vi "PolarizationSimulation_Final.vi"() -> ()   [LabVIEW 2020]
uses:
  Integrated ANN/Sub-VIs/Adam_data.ctl
  <vilib>/Utility/xml.llb/Read From XML File(string).vi
  <vilib>/Utility/xml.llb/Write to XML File(string).vi
  <vilib>/Analysis/NI_AALBase.lvlib
panel:
  out "NN Graph":cluster{dbl[], dbl[]}(graph)
  in  "Regularization":T1
  in  "Batch Size":i16
  out "NN Loss":dbl(graph)
  in  "Loss Function":enum16{"MSE", "MAE"}(ring)
  in  "Parameters File Path":path
  out "NN Error":dbl
  in  "Training?":bool
  out "NN Output":dbl
  in  "Speed\nMultiplier":dbl=1.0
  in  "AFP On":bool
  in  "AFP Efficiency":dbl=0.9 min=0.0 max=1.0 step=0.01
  in  "AFP Control":cluster{i32, i32}(slide)={200, 230} scale=0.0..500.0
  out "lower R-value AFP":dbl
  out "upper R-value AFP":dbl
  in  "STOP":bool
  in  "Microwave Power":dbl=1.0
  in  "Lower Fit\nParameter":dbl=-3.6
  in  "Upper Fit\nParameter":dbl=3.6
  in  "Std Dev Noise":dbl step=0.0001
  out "lower R-value":dbl
  out "upper R-value":dbl
  in  "RF Control":cluster{i32, i32}(slide)={200, 230} scale=0.0..500.0
  out "p":dbl format="%_4g"
  out "r":dbl
  in  "Saturation\nPolarization":dbl=0.8 min=0.0 max=0.99 step=0.01
  out "Reimann \nsum of Q":dbl format="%_4g"
  out "Corrected Data (Q)":cluster{dbl[], dbl[]}(graph)
  in  "Select Target Type":u16(ring)=2 items=["Test Case", "Deuteron"]
  in  "Reset":bool
  out "Total Polarization (P)":cluster{dbl, dbl}(graph)
  in  "Spin Manipulation\nPower Factor":dbl=0.005
  in  "Decay Spin\nManipulation":bool
  out "Reimann\nsum of P":dbl format="%_4g"
  out "Corrected Data (P)":cluster{dbl[], dbl[]}[](graph)
  out "Signal and Fit (P)":cluster{dbl[], "Best Polynomial Fit":dbl[]}[](graph)
  in  "Positive\nPolarization":bool
  in  "Microwave on":bool
  # "Neural Network"
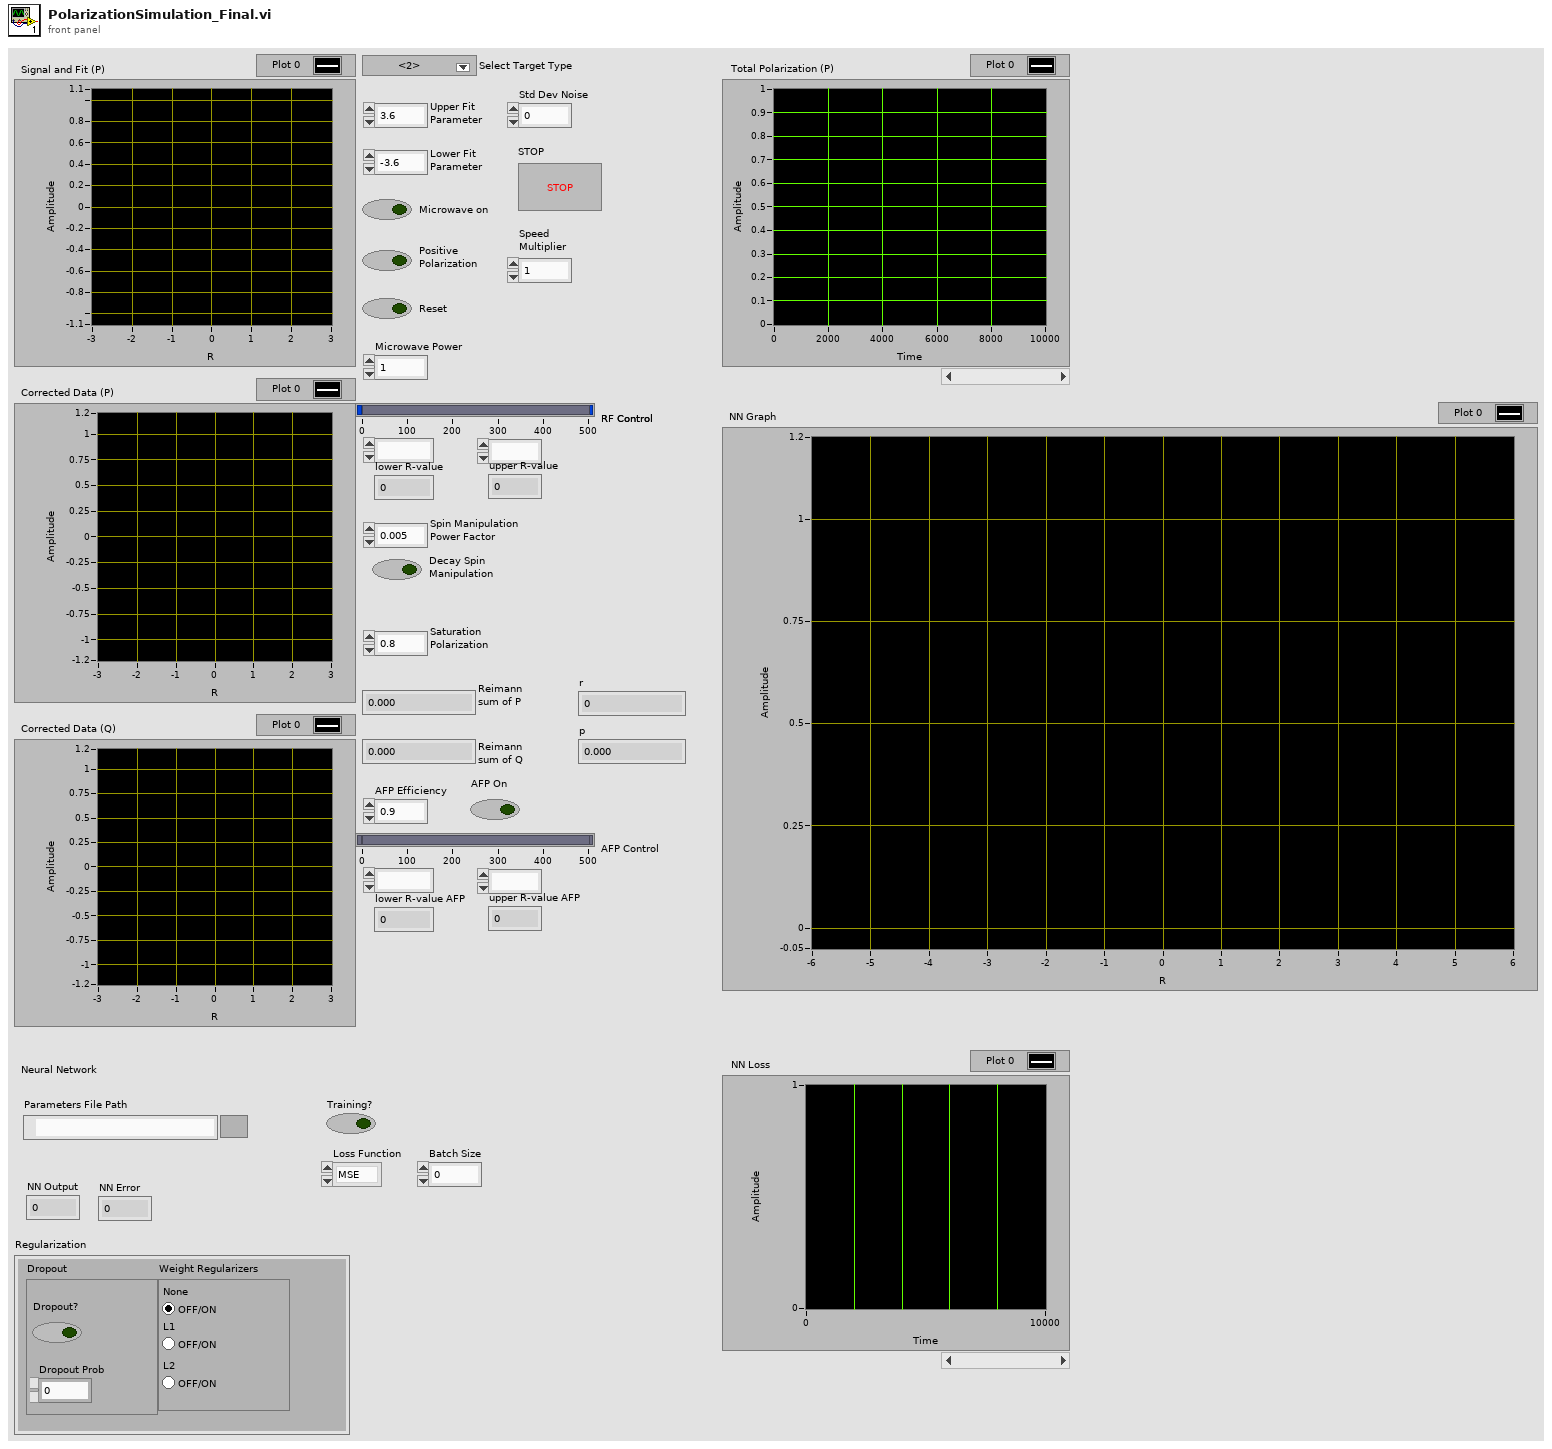
[diagram p1: front panel]
types:
  T1 = cluster{"Dropout":cluster{"Dropout?":bool, "Dropout Prob":dbl}, "Weight Regularizers":enum32{"None", "L1", "L2"}}
  T2 = typedef "Adam_data.ctl" = cluster{"Mw Moments":cluster{"3 ":dbl[], "2":dbl[][], "1":dbl[][]}, "Vw Moments":cluster{"3":dbl[], "2":dbl[][], "1":dbl[][]}, "Mb Moments":cluster{"3":dbl, "2":dbl[], "1":dbl[]}, "Vb Moments":cluster{"3":dbl, "2":dbl[], "1":dbl[]}}
  T3 = cluster{cluster{dbl[][], dbl[]}, cluster{dbl[][], dbl[]}, cluster{dbl[], dbl}}
  T4 = cluster{cluster{"Updated Weights":dbl[][], "Updated Biases":dbl[]}, cluster{"Updated Weights":dbl[][], "Updated Biases":dbl[]}, cluster{"Updated Weights":dbl[], "Updated Biases":dbl}}
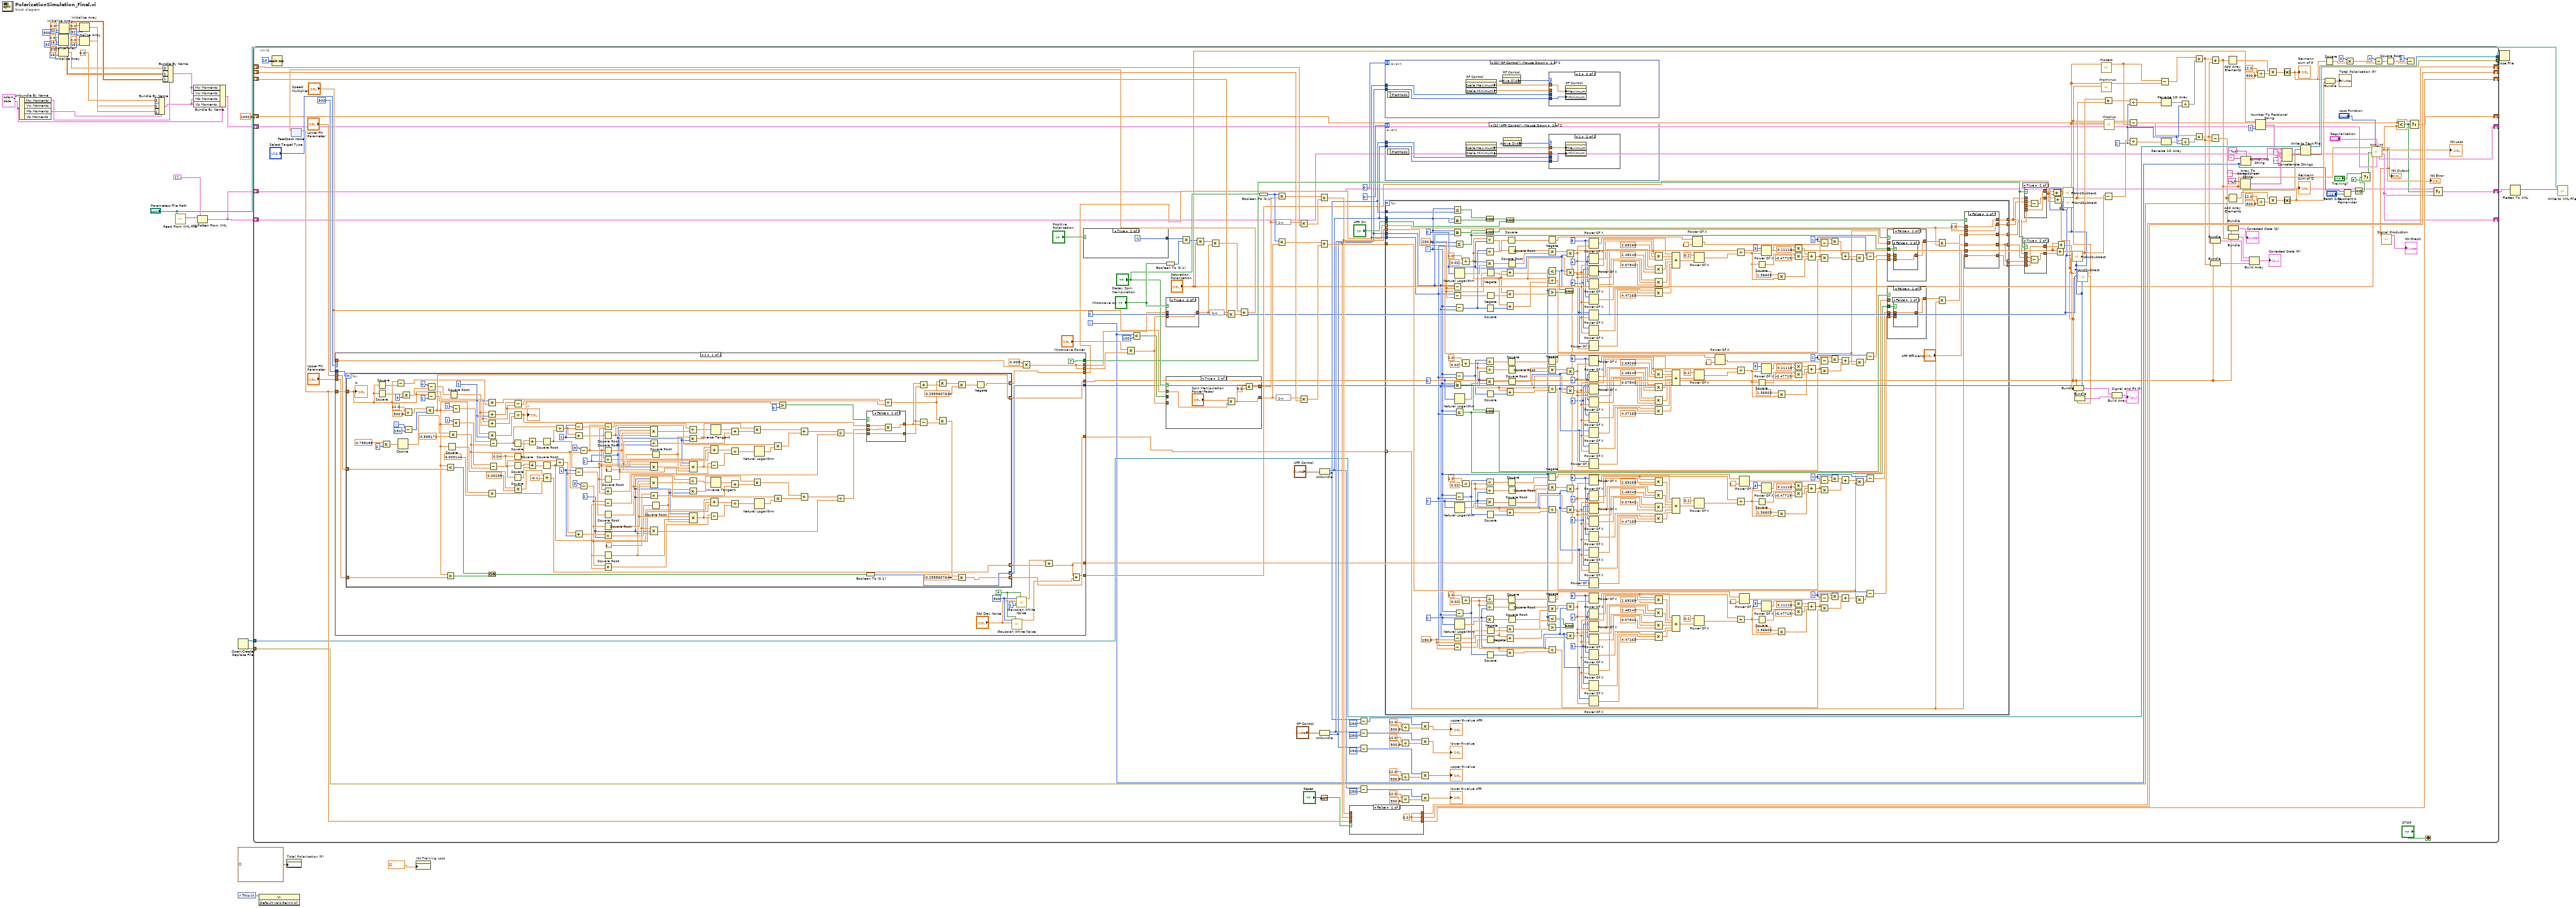
[diagram p0: block diagram]
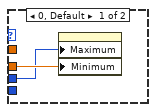
[diagram p2: hidden frame]
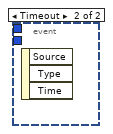
[diagram p3: hidden frame]
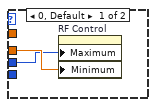
[diagram p4: hidden frame]
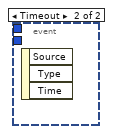
[diagram p5: hidden frame]
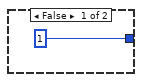
[diagram p6: hidden frame]
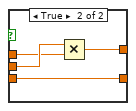
[diagram p7: hidden frame]
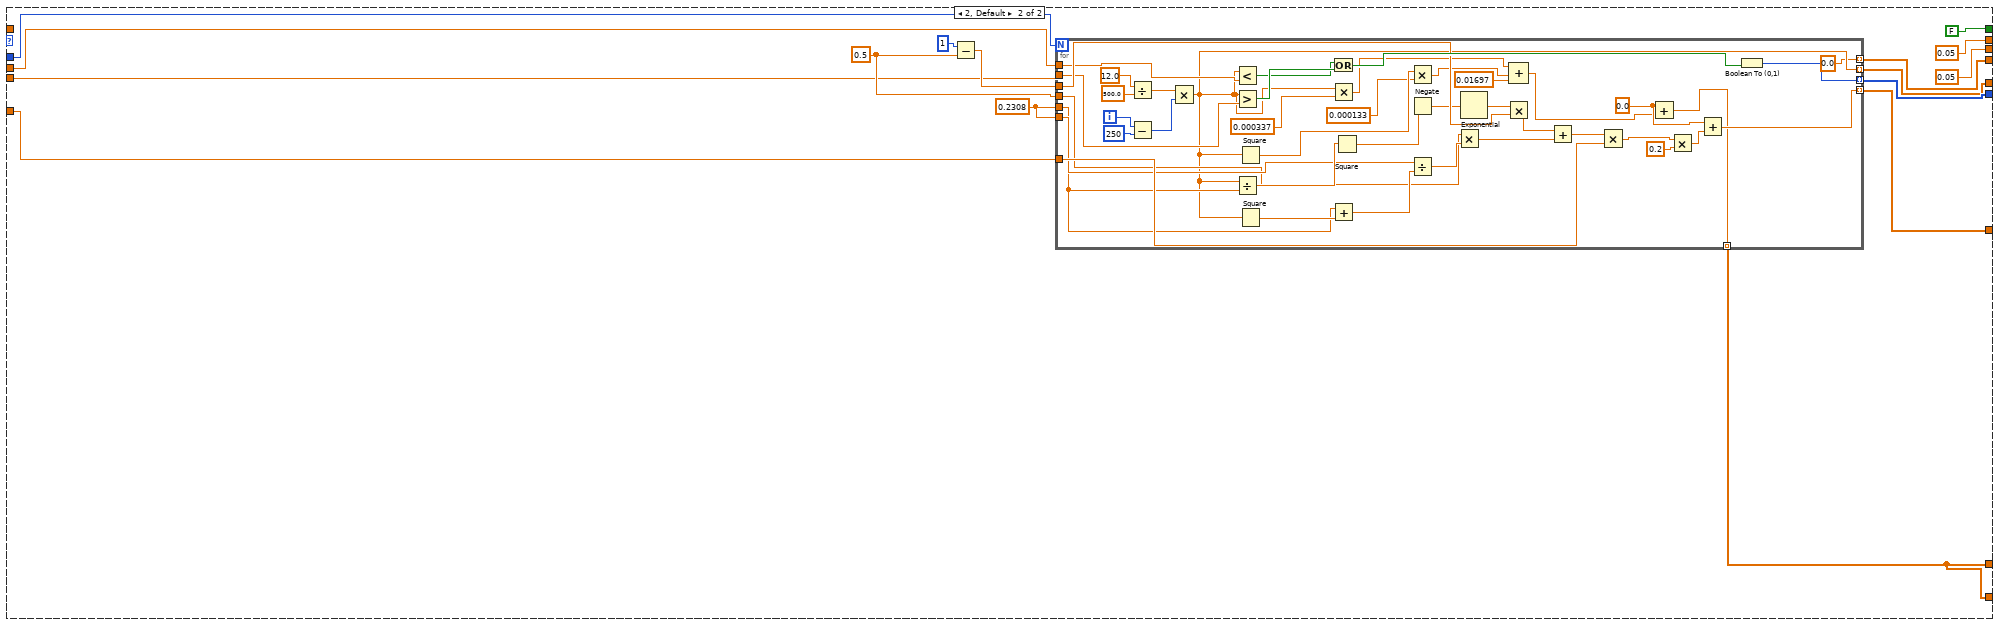
[diagram p8: hidden frame]
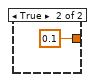
[diagram p10: hidden frame]
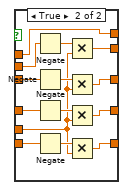
[diagram p15: hidden frame]
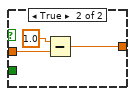
[diagram p17: hidden frame]
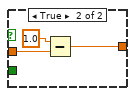
[diagram p19: hidden frame]
diagram:
  w7 = T2 {"Mw Moments"={"3 "=[], "2"=[], "1"=[]}, "Vw Moments"={"3"=[], "2"=[], "1"=[]}, "Mb Moments"={"3"=0.0, "2"=[], "1"=[]}, "Vb Moments"={"3"=0.0, "2"=[], "1"=[]}} ("Adam Data In")
  n1 = Unbundle By Name(w7) -> ("Mw Moments"=w9:cluster{"3 ":dbl[], "2":dbl[][], "1":dbl[][]}, "Mb Moments"=w8:cluster{"3":dbl, "2":dbl[], "1":dbl[]})  [unwired: 2 out]
  n2 = Initialize Array(0.0 ("element"), 16 ("dimension size"), 32 ("dimension size")) -> (w14:dbl[][])
  n3 = Initialize Array(0.0 ("element"), 16 ("dimension size")) -> (w13:dbl[])
  n4 = Initialize Array(0.0 ("element"), 32 ("dimension size"), 500 ("dimension size")) -> (w15:dbl[][])
  n5 = Initialize Array(0.0 ("element"), 16 ("dimension size")) -> (w11:dbl[])
  n6 = Initialize Array(0.0 ("element"), 32 ("dimension size")) -> (w12:dbl[])
  n7 = Bundle By Name(cluster=w8, "3"=0.0 ("element"), "2"=w11, "1"=w12) -> (w5:cluster{"3":dbl, "2":dbl[], "1":dbl[]})
  n8 = Bundle By Name(cluster=w9, "3"=w13, "2"=w14, "1"=w15) -> (w6:cluster{"3 ":dbl[], "2":dbl[][], "1":dbl[][]})
  n9 = call-poly <vilib>:"Read From XML File.vi"("XML File Path"="Parameters File Path") -> ("XML Elements"=w32:string)  [unwired: 8 in, 2 out]
  n10 = Bundle By Name(cluster=w7, "Mw Moments"=w6, "Vw Moments"=w6, "Mb Moments"=w5, "Vb Moments"=w5) -> (w4:T2)
  n11 = Unflatten From XML(xml string=w32, type=T3 {{[], []}, {[], []}, {[], 0.0}}) -> (value=w3:T3)  [unwired: 1 in, 1 out]
  n12 = Open/Create/Replace File() -> (refnum out=w36:refnum<file>, error out=w35:errorcluster)  [unwired: 6 in, 1 out]
  n13 = control-ref of="This VI"() -> (w38:refnum<vi>)
  n14 = while {
    shift-right: [w213] -> _
    shift-left: _ -> [w220]
    shift-right: [w212] -> _
    shift-left: _ -> [w195]
    shift-right: [w190] -> _
    shift-left: _ -> [w189]
    tunnel: w36 -> [w122]
    tunnel: w35 -> [w121]
    tunnel: [w120] -> w34
    tunnel: [w119] -> w33
    shift-right: [w44] -> _
    shift-left: w3 -> [w59]
    shift-right: [w57] -> _
    shift-left: w4 -> [w56]
    shift-right: [w48] -> _
    shift-left: 1000.0 ("Error") -> [w47]
    shift-right: [w43] -> w2
    shift-left: w3 -> [w42]
    i -> [w55]
    stop <- "STOP" stop-if-true
    w172 = 2
    w68 = 2
    n15 = Wait (ms)(milliseconds to wait=10) -> ()  [unwired: 1 out]
    n16 = feedback #1() -> (w199:dbl)  [unwired: 1 in]
    n17 = case shown="1" "Select Target Type" {
      tunnel: [w255 0.05 ("Growth Constant")] -> w204
      tunnel: [w255 0.05 ("Decay Constant")] -> w203
      tunnel: 500 -> [w264 w422]
      tunnel: w199 -> [w267 w421]
      tunnel: "Upper Fit\nParameter" -> [w265 w419]
      tunnel: "Lower Fit\nParameter" -> [w266 w420]
      tunnel: [w262 w417] -> w67
      tunnel: [w252 w416] -> w82
      tunnel: [w263 w418] -> w66
      tunnel: [TRUE FALSE] -> w183
      tunnel: [w253 w412] -> w81
      tunnel: "Speed\nMultiplier" -> [w254 _]
      tunnel: [w248 w411] -> w80
      tunnel: [w250 w411] -> w79
      frame 1 {
        w257 = FALSE
        w259 = 500
        n18 = for {
          N: w264 -> [_]
          tunnel: [w298] -> w262 mode=indexing
          tunnel: [w387] -> w263 mode=indexing
          tunnel: w265 -> [w386]
          tunnel: w266 -> [w385]
          tunnel: [w270] -> w252 mode=indexing
          tunnel: w267 -> [w271]
          tunnel: [w269] -> w253 mode=indexing
          tunnel: [w268] -> w251 mode=indexing
          i -> [w363]
          w285 = 2
          w324 = 1
          w328 = 3.141592653589793
          w322 = 2
          w307 = 0.04
          w360 = 1
          w365 = 3.141592653589793
          w358 = 2
          n19 = Square(x=w271) -> (x^2=w288:dbl)
          n20 = Square(x=w271) -> (x^2=w314:dbl)
          n21 = Multiply(x=0.758188, y=2) -> (x*y=w302:dbl)
          n22 = Subtract(x=w271, y=w288) -> (x-y=w287:dbl)
          n23 = Cosine(x=w302) -> (cos(x)=w305:dbl)
          n24 = Multiply(x=w314, y=3) -> (x*y=w313:dbl)
          n25 = Divide(x=12.0, y=500.0) -> (x/y=w401:dbl)
          n26 = Subtract(x=w363, y=250) -> (x-y=w400:i32)
          n27 = Multiply(x=w401, y=w400) -> (x*y=w298:dbl)
          n28 = Subtract(x=4, y=w313) -> (x-y=w311:dbl)
          n29 = Subtract(x=w271, y=1) -> (x-y=w309:dbl)
          n30 = Less?(x=w298, y=w385) -> (x < y?=w390:bool)
          n31 = Greater?(x=w298, y=w386) -> (0:w389:bool)
          n32 = Square(x=w298) -> (x^2=w300:dbl)
          n33 = Multiply(x=w305, y=0.558171) -> (x*y=w306:dbl)
          n34 = Square Root(x=w311) -> (sqrt(x)=w286:dbl)
          n35 = Subtract(x=1, y=w298) -> (x-y=w395:dbl)
          n36 = Add(x=1, y=w298) -> (x+y=w352:dbl)
          n37 = Multiply(x=w285, y=w287) -> (x*y=w283:dbl)
          n38 = Add(x=w286, y=w285) -> (x+y=w284:dbl)
          n39 = Add(x=w271, y=w286) -> (x+y=w310:dbl)
          n40 = Multiply(x=w309, y=w285) -> (x*y=w293:dbl)
          n41 = Multiply(x=w298, y=0.000144) -> (x*y=w295:dbl)
          n42 = Or(x=w390, y=w389) -> (x .or. y?=w388:bool)
          n43 = Subtract(x=w395, y=w306) -> (x-y=w391:dbl)
          n44 = Subtract(x=w352, y=w306) -> (x-y=w348:dbl)
          n45 = Square(x=w391) -> (x^2=w394:dbl)
          n46 = Square(x=w307) -> (x^2=w393:dbl)
          n47 = Square(x=w307) -> (x^2=w350:dbl)
          n48 = Square(x=w348) -> (x^2=w351:dbl)
          n49 = Subtract(x=w284, y=w271) -> (x-y=w282:dbl)
          n50 = Divide(x=w310, y=w293) -> (x/y=w289:dbl)
          "r" <- w289
          n51 = Multiply(x=w300, y=0.00295) -> (x*y=w299:dbl)
          n52 = Add(x=w393, y=w394) -> (x+y=w392:dbl)
          n53 = Add(x=w350, y=w351) -> (x+y=w349:dbl)
          n54 = Square Root(x=w392) -> (sqrt(x)=w355:dbl)
          n55 = Square Root(x=w349) -> (sqrt(x)=w319:dbl)
          n56 = Compound Arithmetic op=ADD(w299, -0.1, w295) -> (w268:dbl)
          n57 = Divide(x=w391, y=w355) -> (x/y=w361:dbl)
          n58 = Divide(x=w348, y=w319) -> (x/y=w325:dbl)
          n59 = Subtract(x=w360, y=w361) -> (x-y=w316:dbl)
          n60 = Add(x=w361, y=w360) -> (x+y=w359:dbl)
          n61 = Subtract(x=w324, y=w325) -> (x-y=w317:dbl)
          n62 = Add(x=w325, y=w324) -> (x+y=w323:dbl)
          n63 = Subtract(x=3, y=w306) -> (x-y=w371:dbl)
          n64 = Subtract(x=3, y=w306) -> (x-y=w334:dbl)
          n65 = Subtract(x=w371, y=w355) -> (x-y=w380:dbl)
          n66 = Square Root(x=w316) -> (sqrt(x)=w362:dbl)
          n67 = Square Root(x=w371) -> (sqrt(x)=w374:dbl)
          n68 = Divide(x=w359, y=w358) -> (x/y=w357:dbl)
          n69 = Square Root(x=w355) -> (sqrt(x)=w364:dbl)
          n70 = Add(x=w371, y=w355) -> (x+y=w370:dbl)
          n71 = Subtract(x=w334, y=w319) -> (x-y=w343:dbl)
          n72 = Square Root(x=w317) -> (sqrt(x)=w326:dbl)
          n73 = Square Root(x=w334) -> (sqrt(x)=w337:dbl)
          n74 = Divide(x=w323, y=w322) -> (x/y=w321:dbl)
          n75 = Square Root(x=w319) -> (sqrt(x)=w327:dbl)
          n76 = Add(x=w334, y=w319) -> (x+y=w333:dbl)
          n77 = Divide(x=w365, y=w358) -> (x/y=w382:dbl)
          n78 = Divide(x=w328, y=w322) -> (x/y=w345:dbl)
          n79 = Compound Arithmetic op=MULTIPLY(w358, w364, w374, w362) -> (w379:dbl)
          n80 = Compound Arithmetic op=MULTIPLY(w365, w358, w364) -> (w366:dbl)
          n81 = Compound Arithmetic op=MULTIPLY(w322, w327, w337, w326) -> (w342:dbl)
          n82 = Compound Arithmetic op=MULTIPLY(w328, w322, w327) -> (w329:dbl)
          n83 = Square Root(x=w357) -> (sqrt(x)=w356:dbl)
          n84 = Square Root(x=w321) -> (sqrt(x)=w320:dbl)
          n85 = Divide(x=w380, y=w379) -> (x/y=w378:dbl)
          n86 = Multiply(x=w356, y=w358) -> (x*y=w384:dbl)
          n87 = Divide(x=w343, y=w342) -> (x/y=w341:dbl)
          n88 = Multiply(x=w320, y=w322) -> (x*y=w347:dbl)
          n89 = Compound Arithmetic op=MULTIPLY(w358, w374, w364, w356) -> (w369:dbl)
          n90 = Compound Arithmetic op=MULTIPLY(w322, w337, w327, w320) -> (w332:dbl)
          n91 = Subtract(x=w370, y=w369) -> (x-y=w368:dbl)
          n92 = Subtract(x=w333, y=w332) -> (x-y=w331:dbl)
          n93 = Inverse Tangent(1:w378) -> (0:w383:dbl)
          n94 = Compound Arithmetic op=ADD(w369, w355, w371) -> (w373:dbl)
          n95 = Inverse Tangent(1:w341) -> (0:w346:dbl)
          n96 = Compound Arithmetic op=ADD(w332, w319, w334) -> (w336:dbl)
          n97 = Add(x=w383, y=w382) -> (x+y=w381:dbl)
          n98 = Divide(x=w373, y=w368) -> (x/y=w372:dbl)
          n99 = Add(x=w346, y=w345) -> (x+y=w344:dbl)
          n100 = Divide(x=w336, y=w331) -> (x/y=w335:dbl)
          n101 = Multiply(x=w384, y=w381) -> (x*y=w377:dbl)
          n102 = Multiply(x=w347, y=w344) -> (x*y=w340:dbl)
          n103 = Natural Logarithm(1:w372) -> (0:w375:dbl)
          n104 = Natural Logarithm(1:w335) -> (0:w338:dbl)
          n105 = Multiply(x=w362, y=w375) -> (x*y=w376:dbl)
          n106 = Multiply(x=w326, y=w338) -> (x*y=w339:dbl)
          n107 = Greater?(x=w271, y=0) -> (0:w273:bool)
          n108 = Add(x=w377, y=w376) -> (x+y=w367:dbl)
          n109 = Add(x=w340, y=w339) -> (x+y=w330:dbl)
          n110 = Divide(x=w367, y=w366) -> (x/y=w308:dbl)
          n111 = Divide(x=w330, y=w329) -> (x/y=w275:dbl)
          n112 = Boolean To (0,1)(Boolean=w388) -> (0, 1=w387:i16)
          n113 = case shown="False" w273 {
            tunnel: w308 -> [w405 w410]
            tunnel: [w403 w409] -> w291
            tunnel: w289 -> [w406 w408]
            tunnel: w275 -> [w404 w407]
            tunnel: [w404 w407] -> w274
            frame False {
              n114 = Multiply(x=w406, y=w405) -> (x*y=w403:dbl)
            }
            frame True {
              n115 = Multiply(x=w410, y=w408) -> (x*y=w409:dbl)
            }
          }
          n116 = Divide(x=w283, y=w282) -> (x/y=w281:dbl)
          n117 = Add(x=w291, y=w274) -> (x+y=w292:dbl)
          n118 = Subtract(x=w274, y=w291) -> (x-y=w318:dbl)
          n119 = Multiply(x=w281, y=w292) -> (x*y=w280:dbl)
          n120 = Multiply(x=w281, y=w318) -> (x*y=w279:dbl)
          n121 = Multiply(x=w280, y=0.2955607644) -> (x*y=w278:dbl)
          n122 = Multiply(x=w279, y=0.2955607644) -> (x*y=w270:dbl)
          n123 = Negate(x=w278) -> (-x=w269:dbl)
          "p" <- w271
        }
        n124 = call <vilib>:"Gaussian White Noise.vi"("initialize?"=w257, "standard deviation"="Std Dev Noise", "samples"=w259) -> ("Gaussian noise pattern"=w249:dbl[])  [unwired: 7 in, 1 out]
        n125 = call <vilib>:"Gaussian White Noise.vi"("initialize?"=w257, "seed"=1, "standard deviation"="Std Dev Noise", "samples"=w259) -> ("Gaussian noise pattern"=w247:dbl[])  [unwired: 6 in, 1 out]
        n126 = Multiply(x=0.005, y=w254) -> (x*y=w255:dbl)
        n127 = Add(x=w247, y=w251) -> (x+y=w248:dbl[])
        n128 = Add(x=w248, y=w249) -> (x+y=w250:dbl[])
      }
      frame 2, Default {
        w423 = 0.2308
        w424 = 0.5
        n129 = Subtract(x=1, y=w424) -> (x-y=w426:dbl)
        n130 = for {
          N: w422 -> [_]
          tunnel: w421 -> [w466]
          tunnel: [w432] -> w417 mode=indexing
          tunnel: [w450] -> w416 mode=indexing
          tunnel: [w464] -> w418 mode=indexing
          tunnel: w426 -> [w460]
          tunnel: w423 -> [w458]
          tunnel: w423 -> [w439]
          tunnel: w424 -> [w452]
          tunnel: w419 -> [w447]
          tunnel: w420 -> [w446]
          tunnel: [0.0] -> w412 mode=indexing
          tunnel: [w427] -> w411 mode=indexing
          i -> [w440]
          w451 = 0.0
          n131 = Divide(x=12.0, y=500.0) -> (x/y=w441:dbl)
          n132 = Subtract(x=w440, y=250) -> (x-y=w445:i32)
          n133 = Multiply(x=w441, y=w445) -> (x*y=w432:dbl)
          n134 = Less?(x=w432, y=w446) -> (x < y?=w461:bool)
          n135 = Greater?(x=w432, y=w447) -> (0:w462:bool)
          n136 = Divide(x=w432, y=w439) -> (x/y=w467:dbl)
          n137 = Square(x=w432) -> (x^2=w435:dbl)
          n138 = Square(x=w432) -> (x^2=w457:dbl)
          n139 = Or(x=w461, y=w462) -> (x .or. y?=w463:bool)
          n140 = Multiply(x=w432, y=0.000337) -> (x*y=w434:dbl)
          n141 = Add(x=w439, y=w457) -> (x+y=w459:dbl)
          n142 = Square(x=w467) -> (x^2=w468:dbl)
          n143 = Multiply(x=w435, y=0.000133) -> (x*y=w433:dbl)
          n144 = Negate(x=w468) -> (-x=w449:dbl)
          n145 = Divide(x=w458, y=w459) -> (x/y=w454:dbl)
          n146 = Multiply(x=w452, y=w454) -> (x*y=w453:dbl)
          n147 = Exponential(1:w449) -> (0:w448:dbl)
          n148 = Multiply(x=w448, y=w460) -> (x*y=w456:dbl)
          n149 = Compound Arithmetic op=ADD(w434, w433, 0.01697) -> (w436:dbl)
          n150 = Add(x=w456, y=w453) -> (x+y=w455:dbl)
          n151 = Multiply(x=w455, y=w466) -> (x*y=w465:dbl)
          n152 = Add(x=w451, y=w436) -> (x+y=w427:dbl)
          n153 = Multiply(x=w465, y=0.2) -> (x*y=w438:dbl)
          n154 = Add(x=w451, y=w438) -> (x+y=w450:dbl)
          n155 = Boolean To (0,1)(Boolean=w463) -> (0, 1=w464:i16)
        }
      }
    }
    n156 = case shown="True" "Positive\nPolarization" {
      tunnel: [1 -1] -> w157
      frame False {
      }
      frame True {
      }
    }
    n157 = Multiply(x="Microwave Power", y=w204) -> (x*y=w125:dbl)
    n158 = Less?(x=w55, y=100) -> (x < y?=w215:bool)
    n159 = Boolean To (0,1)(Boolean="Microwave on") -> (0, 1=w222:i16)
    n160 = case shown="True" "Microwave on" {
      tunnel: [w479 w480] -> w207
      tunnel: w125 -> [_ w480]
      tunnel: w203 -> [w479 _]
      frame False {
      }
      frame True {
      }
    }
    n161 = case shown="True" "Decay Spin\nManipulation" {
      tunnel: [w469 w475] -> w216
      tunnel: w125 -> [w471 _]
      tunnel: w215 -> [w470 _]
      tunnel: [w469 w476] -> w197
      tunnel: "Speed\nMultiplier" -> [_ w474]
      frame False {
        n162 = case shown="False" w470 {
          tunnel: [w472 0.1] -> w469
          tunnel: w471 -> [w472 _]
          frame False {
          }
          frame True {
          }
        }
      }
      frame True {
        n163 = Multiply(x="Spin Manipulation\nPower Factor", y=w474) -> (x*y=w475:dbl)
        n164 = Multiply(x=w475, y=3.0) -> (x*y=w476:dbl)
      }
    }
    n165 = Multiply(x=w157, y=w222) -> (x*y=w158:i32)
    n166 = Multiply(x=w158, y="Saturation\nPolarization") -> (x*y=w165:dbl)
    n167 = expression code="1-x"(w207) -> (w223:dbl)
    n168 = Multiply(x=w165, y=w207) -> (x*y=w224:dbl)
    n169 = Multiply(x=w223, y=w220) -> (x*y=w225:dbl)
    n170 = Add(x=w224, y=w225) -> (x+y=w202:dbl)
    n171 = feedback-in #1(w202) -> ()
    n172 = Boolean To (0,1)(Boolean="Decay Spin\nManipulation") -> (0, 1=w198:i16)
    n173 = expression code="1-x"(w197) -> (w196:dbl)
    n174 = expression code="1-x"(w216) -> (w217:dbl)
    n175 = Multiply(x=w198, y=w197) -> (x*y=w193:dbl)
    n176 = Multiply(x=w198, y=w216) -> (x*y=w218:dbl)
    n177 = Multiply(x=w196, y=w189) -> (x*y=w194:dbl)
    n178 = Multiply(x=w217, y=w195) -> (x*y=w219:dbl)
    n179 = Add(x=w193, y=w194) -> (x+y=w191:dbl)
    n180 = Add(x=w218, y=w219) -> (x+y=w211:dbl)
    n181 = Not(x="Reset") -> (.not. x?=w210:bool)
    n182 = Unbundle("AFP Control") -> (w89:i32, w88:i32)
    n183 = Unbundle("RF Control") -> (w128:i32, w127:i32)
    n184 = case shown="False" w210 {
      tunnel: [w493 w496] -> w213
      tunnel: w199 -> [_ w496]
      tunnel: [w493 w495] -> w212
      tunnel: w211 -> [_ w495]
      tunnel: w191 -> [_ w494]
      tunnel: [w493 w494] -> w190
      frame False {
        w493 = 0.0
      }
      frame True {
      }
    }
    n185 = Subtract(x=w88, y=250) -> (x-y=w95:i32)
    n186 = Subtract(x=w128, y=250) -> (x-y=w134:i32)
    n187 = Subtract(x=w127, y=250) -> (x-y=w137:i32)
    n188 = Subtract(x=w89, y=250) -> (x-y=w92:i32)
    n189 = event shown="[0] \"RF Control\": Mouse Down" {
      selector: _ -> [_ _]
      dyn-events: _ -> [_ _]
      timeout: 0 -> [_ _]
      tunnel: w128 -> [w237 _]
      tunnel: w127 -> [w236 _]
      event "RF Control": Mouse Down {
        n190 = event-data() -> ()  [unwired: 1 in, 1 out]
        n191 = property on="RF Control" class="Slide (strict)"() -> ("Scale.Maximum"=w238:dbl, "Scale.Minimum"=w239:dbl)  [unwired: 2 in, 2 out]
        n192 = property on="RF Control" class="Slide (strict)"() -> ("Active Slider"=w240:i32)  [unwired: 2 in, 2 out]
        n193 = case shown="1" w240 {
          tunnel: w239 -> [w242 _]
          tunnel: w236 -> [w241 _]
          tunnel: w238 -> [_ w244]
          tunnel: w237 -> [_ w243]
          frame 0, Default {
            n194 = property on="RF Control" class="Slide (strict)"("Maximum"=w241, "Minimum"=w242) -> ()  [unwired: 2 in, 2 out]
          }
          frame 1 {
            n195 = property on="RF Control" class="Slide (strict)"("Maximum"=w244, "Minimum"=w243) -> ()  [unwired: 2 in, 2 out]
          }
        }
      }
      event Timeout {
        n196 = event-data() -> ()  [unwired: 1 in, 3 out]
      }
    }
    n197 = event shown="[0] \"AFP Control\": Mouse Down" {
      selector: _ -> [_ _]
      dyn-events: _ -> [_ _]
      timeout: 0 -> [_ _]
      tunnel: w89 -> [w228 _]
      tunnel: w88 -> [w227 _]
      event "AFP Control": Mouse Down {
        n198 = event-data() -> ()  [unwired: 1 in, 1 out]
        n199 = property on="AFP Control" class="Slide (strict)"() -> ("Scale.Maximum"=w229:dbl, "Scale.Minimum"=w230:dbl)  [unwired: 2 in, 2 out]
        n200 = property on="AFP Control" class="Slide (strict)"() -> ("Active Slider"=w231:i32)  [unwired: 2 in, 2 out]
        n201 = case shown="1" w231 {
          tunnel: w230 -> [w233 _]
          tunnel: w227 -> [w232 _]
          tunnel: w229 -> [_ w235]
          tunnel: w228 -> [_ w234]
          frame 0, Default {
            n202 = property on="AFP Control" class="Slide (strict)"("Maximum"=w232, "Minimum"=w233) -> ()  [unwired: 2 in, 2 out]
          }
          frame 1 {
            n203 = property on="AFP Control" class="Slide (strict)"("Maximum"=w235, "Minimum"=w234) -> ()  [unwired: 2 in, 2 out]
          }
        }
      }
      event Timeout {
        n204 = event-data() -> ()  [unwired: 1 in, 3 out]
      }
    }
    n205 = for {
      tunnel: w82 -> [w509] mode=indexing
      tunnel: w211 -> [w661]
      tunnel: w127 -> [w519]
      tunnel: w128 -> [w518]
      tunnel: [w505] -> w201 mode=indexing
      tunnel: [w506] -> w192 mode=indexing
      tunnel: [w506] -> w200 mode=indexing
      tunnel: w81 -> [w498] mode=indexing
      tunnel: w191 -> [w517]
      tunnel: [w497] -> w187 mode=indexing
      tunnel: [w504] -> w177 mode=indexing
      tunnel: w89 -> [w513]
      tunnel: w88 -> [w512]
      tunnel: "AFP On" -> [w501]
      tunnel: [w500] -> w86 mode=indexing
      i -> [w511]
      w521 = 250.0
      w560 = 5
      w558 = 4
      w557 = 3
      w538 = 1
      w539 = 2
      w621 = 5
      w619 = 4
      w618 = 3
      w598 = 1
      w599 = 2
      w655 = 250.0
      w696 = 5
      w694 = 4
      w693 = 3
      w674 = 1
      w675 = 2
      w757 = 5
      w755 = 4
      w754 = 3
      w734 = 1
      w735 = 2
      n206 = Less Or Equal?(x=w511, y=w512) -> (x <= y?=w514:bool)
      n207 = Greater Or Equal?(x=w511, y=w513) -> (x >= y?=w515:bool)
      n208 = Greater Or Equal?(x=w511, y=w518) -> (x >= y?=w594:bool)
      n209 = Subtract(x=w518, y=w521) -> (x-y=w525:dbl)
      n210 = Subtract(x=w519, y=w521) -> (x-y=w526:dbl)
      n211 = Greater Or Equal?(x=w511, y=w518) -> (x >= y?=w730:bool)
      n212 = Subtract(x=w518, y=w655) -> (x-y=w659:dbl)
      n213 = Subtract(x=w519, y=w655) -> (x-y=w660:dbl)
      n214 = Less Or Equal?(x=w511, y=w519) -> (x <= y?=w531:bool)
      n215 = Natural Logarithm(1:w599) -> (0:w634:dbl)
      n216 = Subtract(x=w511, y=w518) -> (x-y=w607:i32)
      n217 = Subtract(x=w511, y=w519) -> (x-y=w546:i32)
      n218 = Natural Logarithm(1:w539) -> (0:w573:dbl)
      n219 = Less Or Equal?(x=w511, y=w519) -> (x <= y?=w666:bool)
      n220 = Subtract(x=w511, y=w519) -> (x-y=w682:i32)
      n221 = Natural Logarithm(1:w675) -> (0:w709:dbl)
      n222 = Subtract(x=w511, y=w518) -> (x-y=w743:i32)
      n223 = Natural Logarithm(1:w735) -> (0:w770:dbl)
      n224 = Divide(x=1.0, y=0.02) -> (x/y=w603:dbl)
      n225 = Divide(x=1.0, y=0.02) -> (x/y=w543:dbl)
      n226 = Divide(x=1.0, y=0.02) -> (x/y=w679:dbl)
      n227 = Divide(x=1.0, y=0.02) -> (x/y=w739:dbl)
      n228 = And(x=w514, y=w515) -> (x .and. y?=w503:bool)
      n229 = And(x=w594, y=w531) -> (x .and. y?=w532:bool)
      n230 = Divide(x=w603, y=w599) -> (x/y=w632:dbl)
      n231 = Divide(x=w607, y=w603) -> (x/y=w611:dbl)
      n232 = Multiply(x=w599, y=w634) -> (x*y=w635:dbl)
      n233 = Divide(x=w546, y=w543) -> (x/y=w550:dbl)
      n234 = Divide(x=w543, y=w539) -> (x/y=w571:dbl)
      n235 = Multiply(x=w539, y=w573) -> (x*y=w574:dbl)
      n236 = And(x=w730, y=w666) -> (x .and. y?=w668:bool)
      n237 = Divide(x=w682, y=w679) -> (x/y=w686:dbl)
      n238 = Divide(x=w679, y=w675) -> (x/y=w707:dbl)
      n239 = Multiply(x=w675, y=w709) -> (x*y=w710:dbl)
      n240 = Divide(x=w743, y=w739) -> (x/y=w747:dbl)
      n241 = Divide(x=w739, y=w735) -> (x/y=w768:dbl)
      n242 = Multiply(x=w735, y=w770) -> (x*y=w771:dbl)
      n243 = Square(x=w607) -> (x^2=w608:i32)
      n244 = Square(x=w546) -> (x^2=w547:i32)
      n245 = Square(x=w682) -> (x^2=w683:i32)
      n246 = Square(x=w743) -> (x^2=w744:i32)
      n247 = Negate(x=w525) -> (-x=w524:dbl)
      n248 = Negate(x=w526) -> (-x=w522:dbl)
      n249 = Negate(x=w659) -> (-x=w658:dbl)
      n250 = Negate(x=w660) -> (-x=w656:dbl)
      n251 = Add(x=w521, y=w524) -> (x+y=w523:dbl)
      n252 = Add(x=w521, y=w522) -> (x+y=w520:dbl)
      n253 = Add(x=w603, y=w608) -> (x+y=w609:dbl)
      n254 = Add(x=w543, y=w547) -> (x+y=w548:dbl)
      n255 = Add(x=w679, y=w683) -> (x+y=w684:dbl)
      n256 = Add(x=w655, y=w658) -> (x+y=w657:dbl)
      n257 = Add(x=w655, y=w656) -> (x+y=w654:dbl)
      n258 = Add(x=w739, y=w744) -> (x+y=w745:dbl)
      n259 = And(x=w503, y=w501) -> (x .and. y?=w502:bool)
      n260 = Square(x=w611) -> (x^2=w613:dbl)
      n261 = Square(x=w550) -> (x^2=w552:dbl)
      n262 = Square(x=w686) -> (x^2=w688:dbl)
      n263 = Square(x=w747) -> (x^2=w749:dbl)
      n264 = Square Root(x=w632) -> (sqrt(x)=w633:dbl)
      n265 = Square Root(x=w635) -> (sqrt(x)=w636:dbl)
      n266 = Square Root(x=w571) -> (sqrt(x)=w572:dbl)
      n267 = Square Root(x=w574) -> (sqrt(x)=w575:dbl)
      n268 = Square Root(x=w707) -> (sqrt(x)=w708:dbl)
      n269 = Square Root(x=w710) -> (sqrt(x)=w711:dbl)
      n270 = Square Root(x=w768) -> (sqrt(x)=w769:dbl)
      n271 = Square Root(x=w771) -> (sqrt(x)=w772:dbl)
      n272 = Negate(x=w613) -> (-x=w612:dbl)
      n273 = Multiply(x=w633, y=w636) -> (x*y=w627:dbl)
      n274 = Less?(x=w511, y=w523) -> (x < y?=w528:bool)
      n275 = Divide(x=w603, y=w609) -> (x/y=w606:dbl)
      n276 = Greater?(x=w511, y=w520) -> (0:w527:bool)
      n277 = Negate(x=w552) -> (-x=w551:dbl)
      n278 = Multiply(x=w572, y=w575) -> (x*y=w566:dbl)
      n279 = Divide(x=w543, y=w548) -> (x/y=w533:dbl)
      n280 = Negate(x=w688) -> (-x=w687:dbl)
      n281 = Multiply(x=w708, y=w711) -> (x*y=w702:dbl)
      n282 = Divide(x=w679, y=w684) -> (x/y=w669:dbl)
      n283 = Negate(x=w749) -> (-x=w748:dbl)
      n284 = Multiply(x=w769, y=w772) -> (x*y=w763:dbl)
      n285 = Less?(x=w511, y=w657) -> (x < y?=w663:bool)
      n286 = Greater?(x=w511, y=w654) -> (0:w662:bool)
      n287 = Divide(x=w739, y=w745) -> (x/y=w742:dbl)
      n288 = And(x=w528, y=w527) -> ()  [unwired: 1 out]
      n289 = And(x=w663, y=w662) -> ()  [unwired: 1 out]
      n290 = Multiply(x=w627, y=w599) -> (x*y=w651:dbl)
      n291 = Multiply(x=w599, y=w603) -> (x*y=w645:dbl)
      n292 = Multiply(x=w566, y=w539) -> (x*y=w590:dbl)
      n293 = Multiply(x=w539, y=w543) -> (x*y=w584:dbl)
      n294 = Multiply(x=w702, y=w675) -> (x*y=w726:dbl)
      n295 = Multiply(x=w675, y=w679) -> (x*y=w720:dbl)
      n296 = Multiply(x=w763, y=w735) -> (x*y=w787:dbl)
      n297 = Multiply(x=w735, y=w739) -> (x*y=w781:dbl)
      n298 = Power Of X(1:w651, 2:w621) -> (0:w638:dbl)
      n299 = Power Of X(1:w651, 2:w619) -> (0:w644:dbl)
      n300 = Power Of X(1:w651, 2:w618) -> (0:w646:dbl)
      n301 = Power Of X(1:w645, 2:w619) -> (0:w650:dbl)
      n302 = Power Of X(1:w645, 2:w621) -> (0:w639:dbl)
      n303 = Power Of X(1:w645, 2:w599) -> (0:w647:dbl)
      n304 = Power Of X(1:w645, 2:w618) -> (0:w648:dbl)
      n305 = Power Of X(1:w651, 2:w599) -> (0:w649:dbl)
      n306 = Power Of X(1:w590, 2:w560) -> (0:w577:dbl)
      n307 = Power Of X(1:w590, 2:w558) -> (0:w583:dbl)
      n308 = Power Of X(1:w590, 2:w557) -> (0:w585:dbl)
      n309 = Power Of X(1:w584, 2:w558) -> (0:w589:dbl)
      n310 = Power Of X(1:w584, 2:w560) -> (0:w578:dbl)
      n311 = Power Of X(1:w584, 2:w539) -> (0:w586:dbl)
      n312 = Power Of X(1:w584, 2:w557) -> (0:w587:dbl)
      n313 = Power Of X(1:w590, 2:w539) -> (0:w588:dbl)
      n314 = Power Of X(1:w726, 2:w696) -> (0:w713:dbl)
      n315 = Power Of X(1:w726, 2:w694) -> (0:w719:dbl)
      n316 = Power Of X(1:w726, 2:w693) -> (0:w721:dbl)
      n317 = Power Of X(1:w720, 2:w694) -> (0:w725:dbl)
      n318 = Power Of X(1:w720, 2:w696) -> (0:w714:dbl)
      n319 = Power Of X(1:w720, 2:w675) -> (0:w722:dbl)
      n320 = Power Of X(1:w720, 2:w693) -> (0:w723:dbl)
      n321 = Power Of X(1:w726, 2:w675) -> (0:w724:dbl)
      n322 = Power Of X(1:w787, 2:w757) -> (0:w774:dbl)
      n323 = Power Of X(1:w787, 2:w755) -> (0:w780:dbl)
      n324 = Power Of X(1:w787, 2:w754) -> (0:w782:dbl)
      n325 = Power Of X(1:w781, 2:w755) -> (0:w786:dbl)
      n326 = Power Of X(1:w781, 2:w757) -> (0:w775:dbl)
      n327 = Power Of X(1:w781, 2:w735) -> (0:w783:dbl)
      n328 = Power Of X(1:w781, 2:w754) -> (0:w784:dbl)
      n329 = Power Of X(1:w787, 2:w735) -> (0:w785:dbl)
      n330 = Compound Arithmetic op=MULTIPLY(w645, w644, 2.69269) -> (w640:dbl)
      n331 = Compound Arithmetic op=MULTIPLY(w646, w647, 2.48243) -> (w642:dbl)
      n332 = Compound Arithmetic op=MULTIPLY(w651, w650, 0.07842) -> (w641:dbl)
      n333 = Compound Arithmetic op=MULTIPLY(w648, w649, 4.47163) -> (w643:dbl)
      n334 = Compound Arithmetic op=MULTIPLY(w584, w583, 2.69269) -> (w579:dbl)
      n335 = Compound Arithmetic op=MULTIPLY(w585, w586, 2.48243) -> (w581:dbl)
      n336 = Compound Arithmetic op=MULTIPLY(w590, w589, 0.07842) -> (w580:dbl)
      n337 = Compound Arithmetic op=MULTIPLY(w587, w588, 4.47163) -> (w582:dbl)
      n338 = Compound Arithmetic op=MULTIPLY(w720, w719, 2.69269) -> (w715:dbl)
      n339 = Compound Arithmetic op=MULTIPLY(w721, w722, 2.48243) -> (w717:dbl)
      n340 = Compound Arithmetic op=MULTIPLY(w726, w725, 0.07842) -> (w716:dbl)
      n341 = Compound Arithmetic op=MULTIPLY(w723, w724, 4.47163) -> (w718:dbl)
      n342 = Compound Arithmetic op=MULTIPLY(w781, w780, 2.69269) -> (w776:dbl)
      n343 = Compound Arithmetic op=MULTIPLY(w782, w783, 2.48243) -> (w778:dbl)
      n344 = Compound Arithmetic op=MULTIPLY(w787, w786, 0.07842) -> (w777:dbl)
      n345 = Compound Arithmetic op=MULTIPLY(w784, w785, 4.47163) -> (w779:dbl)
      n346 = Compound Arithmetic op=unknown(w638, w640, w642, w641, w639, w643) -> (w600:dbl)
      n347 = Compound Arithmetic op=unknown(w577, w579, w581, w580, w578, w582) -> (w540:dbl)
      n348 = Compound Arithmetic op=unknown(w713, w715, w717, w716, w714, w718) -> (w676:dbl)
      n349 = Compound Arithmetic op=unknown(w774, w776, w778, w777, w775, w779) -> (w736:dbl)
      n350 = Power Of X(1:2.718281828459045, 2:w612) -> (0:w610:dbl)
      n351 = Power Of X(1:w600, 2:0.2) -> (0:w653:dbl)
      n352 = Power Of X(1:w540, 2:0.2) -> (0:w592:dbl)
      n353 = Power Of X(1:w676, 2:0.2) -> (0:w728:dbl)
      n354 = Power Of X(1:w736, 2:0.2) -> (0:w789:dbl)
      n355 = Power Of X(1:2.718281828459045, 2:w551) -> (0:w549:dbl)
      n356 = Divide(x=w645, y=w653) -> (x/y=w637:dbl)
      n357 = Divide(x=w584, y=w592) -> (x/y=w576:dbl)
      n358 = Divide(x=w720, y=w728) -> (x/y=w712:dbl)
      n359 = Divide(x=w781, y=w789) -> (x/y=w773:dbl)
      n360 = Power Of X(1:2.718281828459045, 2:w687) -> (0:w685:dbl)
      n361 = Power Of X(1:2.718281828459045, 2:w748) -> (0:w746:dbl)
      n362 = Square(x=w637) -> (x^2=w631:dbl)
      n363 = Square(x=w576) -> (x^2=w570:dbl)
      n364 = Square(x=w712) -> (x^2=w706:dbl)
      n365 = Square(x=w773) -> (x^2=w767:dbl)
      n366 = Power Of X(1:w637, 2:3) -> (0:w630:dbl)
      n367 = Power Of X(1:w576, 2:3) -> (0:w569:dbl)
      n368 = Power Of X(1:w712, 2:3) -> (0:w705:dbl)
      n369 = Power Of X(1:w773, 2:3) -> (0:w766:dbl)
      n370 = Multiply(x=1.36603, y=w637) -> (x*y=w652:dbl)
      n371 = Multiply(x=1.36603, y=w576) -> (x*y=w591:dbl)
      n372 = Multiply(x=1.36603, y=w712) -> (x*y=w727:dbl)
      n373 = Multiply(x=1.36603, y=w773) -> (x*y=w788:dbl)
      n374 = Multiply(x=w630, y=0.11116) -> (x*y=w629:dbl)
      n375 = Multiply(x=w631, y=-0.47719) -> (x*y=w628:dbl)
      n376 = Multiply(x=w569, y=0.11116) -> (x*y=w568:dbl)
      n377 = Multiply(x=w570, y=-0.47719) -> (x*y=w567:dbl)
      n378 = Multiply(x=w705, y=0.11116) -> (x*y=w704:dbl)
      n379 = Multiply(x=w706, y=-0.47719) -> (x*y=w703:dbl)
      n380 = Multiply(x=w766, y=0.11116) -> (x*y=w765:dbl)
      n381 = Multiply(x=w767, y=-0.47719) -> (x*y=w764:dbl)
      n382 = Compound Arithmetic op=unknown(w629, w628, w652) -> (w604:dbl)
      n383 = Compound Arithmetic op=unknown(w568, w567, w591) -> (w544:dbl)
      n384 = Compound Arithmetic op=unknown(w704, w703, w727) -> (w680:dbl)
      n385 = Compound Arithmetic op=unknown(w765, w764, w788) -> (w740:dbl)
      n386 = Subtract(x=w598, y=w604) -> (x-y=w601:dbl)
      n387 = Multiply(x=w604, y=w606) -> (x*y=w605:dbl)
      n388 = Subtract(x=w538, y=w544) -> (x-y=w541:dbl)
      n389 = Multiply(x=w544, y=w533) -> (x*y=w545:dbl)
      n390 = Subtract(x=w674, y=w680) -> (x-y=w677:dbl)
      n391 = Multiply(x=w680, y=w669) -> (x*y=w681:dbl)
      n392 = Subtract(x=w734, y=w740) -> (x-y=w737:dbl)
      n393 = Multiply(x=w740, y=w742) -> (x*y=w741:dbl)
      n394 = Multiply(x=w610, y=w601) -> (x*y=w602:dbl)
      n395 = Multiply(x=w549, y=w541) -> (x*y=w542:dbl)
      n396 = Multiply(x=w685, y=w677) -> (x*y=w678:dbl)
      n397 = Multiply(x=w746, y=w737) -> (x*y=w738:dbl)
      n398 = Add(x=w602, y=w605) -> (x+y=w597:dbl)
      n399 = Add(x=w542, y=w545) -> (x+y=w537:dbl)
      n400 = Add(x=w678, y=w681) -> (x+y=w673:dbl)
      n401 = Add(x=w738, y=w741) -> (x+y=w733:dbl)
      n402 = Multiply(x=w597, y=w517) -> (x*y=w596:dbl)
      n403 = Multiply(x=w537, y=w517) -> (x*y=w536:dbl)
      n404 = Multiply(x=w673, y=w661) -> (x*y=w672:dbl)
      n405 = Multiply(x=w733, y=w661) -> (x*y=w732:dbl)
      n406 = Subtract(x=w598, y=w596) -> (x-y=w530:dbl)
      n407 = Subtract(x=w538, y=w536) -> (x-y=w529:dbl)
      n408 = Subtract(x=w674, y=w672) -> (x-y=w664:dbl)
      n409 = Subtract(x=w734, y=w732) -> (x-y=w665:dbl)
      n410 = case shown="False" w532 {
        tunnel: [w809 w815] -> w516
        tunnel: w517 -> [_ w816]
        tunnel: w531 -> [w812 _]
        tunnel: w530 -> [w811 _]
        tunnel: w529 -> [w810 _]
        frame False {
          n411 = case shown="False" w812 {
            tunnel: [w813 w814] -> w809
            tunnel: w811 -> [_ w814]
            tunnel: w810 -> [w813 _]
            frame False {
            }
            frame True {
            }
          }
        }
        frame True {
          n412 = Subtract(x=1.0, y=w816) -> (x-y=w815:dbl)
        }
      }
      n413 = case shown="False" w668 {
        tunnel: [w818 w824] -> w667
        tunnel: w661 -> [_ w825]
        tunnel: w666 -> [w821 _]
        tunnel: w665 -> [w820 _]
        tunnel: w664 -> [w819 _]
        frame False {
          n414 = case shown="False" w821 {
            tunnel: [w822 w823] -> w818
            tunnel: w820 -> [_ w823]
            tunnel: w819 -> [w822 _]
            frame False {
            }
            frame True {
            }
          }
        }
        frame True {
          n415 = Subtract(x=1.0, y=w825) -> (x-y=w824:dbl)
        }
      }
      n416 = Multiply(x=w516, y=w498) -> (x*y=w499:dbl)
      n417 = Multiply(x=w667, y=w509) -> (x*y=w508:dbl)
      n418 = case shown="False" w502 {
        tunnel: 0.0 -> [w794 w801]
        tunnel: w509 -> [w793 w808]
        tunnel: w508 -> [w792 w807]
        tunnel: "AFP Efficiency" -> [_ w795]
        tunnel: [w792 w803] -> w506
        tunnel: [w793 w802] -> w505
        tunnel: [w794 w801] -> w504
        tunnel: w499 -> [w791 w800]
        tunnel: [w791 w799] -> w500
        tunnel: w498 -> [w790 w798]
        tunnel: [w790 w796] -> w497
        frame False {
        }
        frame True {
          n419 = Negate(x=w798) -> (-x=w797:dbl)
          n420 = Negate(x=w800) -> (-x=w806:dbl)
          n421 = Negate(x=w807) -> (-x=w805:dbl)
          n422 = Negate(x=w808) -> (-x=w804:dbl)
          n423 = Multiply(x=w797, y=w795) -> (x*y=w796:dbl)
          n424 = Multiply(x=w806, y=w795) -> (x*y=w799:dbl)
          n425 = Multiply(x=w805, y=w795) -> (x*y=w803:dbl)
          n426 = Multiply(x=w804, y=w795) -> (x*y=w802:dbl)
        }
      }
    }
    n427 = Divide(x=12.0, y=500.0) -> (x/y=w103:dbl)
    n428 = Divide(x=12.0, y=500.0) -> (x/y=w141:dbl)
    n429 = Divide(x=12.0, y=500.0) -> (x/y=w145:dbl)
    n430 = Divide(x=12.0, y=500.0) -> (x/y=w99:dbl)
    n431 = Multiply(x=w95, y=w103) -> (x*y=→"upper R-value AFP":dbl)
    n432 = Multiply(x=w134, y=w141) -> (x*y=→"lower R-value":dbl)
    n433 = Multiply(x=w137, y=w145) -> (x*y=→"upper R-value":dbl)
    n434 = Multiply(x=w92, y=w99) -> (x*y=→"lower R-value AFP":dbl)
    n435 = case shown="True" w183 {
      tunnel: w187 -> [_ w486]
      tunnel: w86 -> [w482 w485]
      tunnel: w86 -> [_ w484]
      tunnel: [w482 w484] -> w186
      tunnel: [w481 w483] -> w174
      tunnel: w177 -> [w481 _]
      frame False {
      }
      frame True {
        n436 = Subtract(x=w486, y=w485) -> (x-y=w483:dbl[])
      }
    }
    n437 = case shown="True" w183 {
      tunnel: w201 -> [_ w492]
      tunnel: w192 -> [w488 w491]
      tunnel: w200 -> [_ w490]
      tunnel: [w488 w490] -> w184
      tunnel: [w487 w489] -> w173
      tunnel: w177 -> [w487 _]
      frame False {
      }
      frame True {
        n438 = Subtract(x=w492, y=w491) -> (x-y=w489:dbl[])
      }
    }
    n439 = Add(x=w186, y=w79) -> (x+y=w69:dbl[])
    n440 = Add(x=w174, y=w79) -> (x+y=w71:dbl[])
    n441 = Add(x=w80, y=w173) -> (x+y=w73:dbl[])
    n442 = Add(x=w80, y=w184) -> (x+y=w75:dbl[])
    n443 = call "FitAndSubtract.vi"("Array 4"=w66, "Array 3"=w67, "Numeric"=w68, "Array in"=w69) -> ("Array out"=w70:dbl[])  [unwired: 6 in, 1 out]
    n444 = call "FitAndSubtract.vi"("Array 4"=w66, "Array 3"=w67, "Numeric"=w68, "Array in"=w71) -> ("Array out"=w72:dbl[])  [unwired: 6 in, 1 out]
    n445 = call "FitAndSubtract.vi"("Array 4"=w66, "Array 3"=w67, "Numeric"=w68, "Array in"=w73) -> ("Array out"=w76:dbl[])  [unwired: 6 in, 1 out]
    n446 = Bundle(w67, w75) -> (w226:cluster{dbl[], dbl[]})  [unwired: 1 in]
    n447 = call "FitAndSubtract.vi"("Array 4"=w66, "Array 3"=w67, "Numeric"=w68, "Array in"=w75) -> ("Best Polynomial Fit"=w74:dbl[], "Array out"=w77:dbl[])  [unwired: 6 in]
    n448 = Bundle(w67, "Best Polynomial Fit"=w74) -> (w160:cluster{dbl[], "Best Polynomial Fit":dbl[]})  [unwired: 1 in]
    n449 = call "rhozero.vi"("Array in"=w70) -> ("Array out"=w181:dbl[])  [unwired: 10 in]
    n450 = call "rhominus.vi"("Array"=w77, "Array 2"=w70) -> ("Array 3"=w180:dbl[])  [unwired: 9 in]
    n451 = Add(x=w76, y=w72) -> (x+y=w175:dbl[])
    n452 = Subtract(x=w76, y=w72) -> (x-y=w176:dbl[])
    n453 = call "rhoplus.vi"("Array 3"=w70, "Array in"=w77) -> ("Array out"=w182:dbl[])  [unwired: 9 in]
    n454 = Build Array(w226, w160) -> (→"Signal and Fit (P)":cluster{dbl[], "Best Polynomial Fit":dbl[]}[])
    n455 = Divide(x=w175, y=w172) -> (x/y=w171:dbl[])
    n456 = Subtract(x=w182, y=w181) -> (x-y=w169:dbl[])
    n457 = Divide(x=w176, y=w172) -> (x/y=w170:dbl[])
    n458 = Subtract(x=w181, y=w180) -> (x-y=w168:dbl[])
    n459 = Reverse 1D Array(array=w171) -> (reversed array=w179:dbl[])
    n460 = Reverse 1D Array(array=w170) -> (reversed array=w178:dbl[])
    n461 = Divide(x=w179, y=w172) -> (x/y=w83:dbl[])
    n462 = Divide(x=w178, y=w172) -> (x/y=w84:dbl[])
    n463 = Add(x=w168, y=w83) -> (x+y=w166:dbl[])
    n464 = Add(x=w169, y=w84) -> (x+y=w167:dbl[])
    n465 = Subtract(x=w167, y=w166) -> (x-y=w154:dbl[])
    n466 = Add(x=w166, y=w167) -> (x+y=w61:dbl[])
    n467 = Bundle(w67, w167) -> (w161:cluster{dbl[], dbl[]})  [unwired: 1 in]
    n468 = Bundle(w67, w166) -> (w162:cluster{dbl[], dbl[]})  [unwired: 1 in]
    n469 = Add Array Elements(numeric array=w61) -> (sum=w156:dbl)
    n470 = Add Array Elements(numeric array=w154) -> (sum=w155:dbl)
    n471 = Bundle(w67, w154) -> (→"Corrected Data (Q)":cluster{dbl[], dbl[]})  [unwired: 1 in]
    n472 = Bundle(w67, w61) -> (w163:cluster{dbl[], dbl[]})  [unwired: 1 in]
    n473 = Array To Spreadsheet String(delimiter (Tab)=",", array=w61, 3:"%f") -> (spreadsheet string=w65:string)
    n474 = Format Into String(format string="%d", initial string="", w55) -> (resulting string=w116:string)  [unwired: 1 in, 1 out]
    n475 = Build Array(w163, w161, w162) -> (→"Corrected Data (P)":cluster{dbl[], dbl[]}[])
    n476 = Number To Fractional String(number="Saturation\nPolarization", precision (6)=i16 2) -> (F-format string=w63:string)  [unwired: 2 in]
    n477 = Divide(x=12.0, y=500.0) -> (x/y=w152:dbl)
    n478 = Divide(x=12.0, y=500.0) -> (x/y=w146:dbl)
    n479 = Multiply(x=w156, y=w152) -> (x*y=w153:dbl)
    n480 = Multiply(x=w155, y=w146) -> (x*y=w149:dbl)
    n481 = Absolute Value(x=w153) -> (abs(x)=w106:dbl)
    "Reimann\nsum of P" <- w106
    n482 = Concatenate Strings(w116, ",", w63, ",", w65) -> (w113:string)
    n483 = Absolute Value(x=w149) -> (abs(x)=w133:dbl)
    "Reimann \nsum of Q" <- w133
    n484 = Write to Text File(file (use dialog)=w122, text=w113, error in=w121) -> (refnum out=w120:refnum<file>, error out=w119:errorcluster)  [unwired: 1 in, 1 out]
    n485 = Square(x=w106) -> (x^2=w104:dbl)
    n486 = Bundle(w106, w133) -> (→"Total Polarization (P)":cluster{dbl, dbl})  [unwired: 1 in]
    n487 = Quotient & Remainder(x=w55, y="Batch Size") -> (x-y*floor(x/y)=w53:i32)  [unwired: 1 out]
    n488 = Multiply(x=3, y=w104) -> (x*y=w108:dbl)
    n489 = Equal To 0?(x=w53) -> (x = 0?=w52:bool)
    n490 = Select(t="Training?", s=w52, f=FALSE) -> (s? t:f=w49:bool)
    n491 = call "Ann_int.vi"("Data"=w61, "Loss Function"="Loss Function", "Regularization"="Regularization", "Target"="Saturation\nPolarization", "Training?"=w49, "Parameters"=w59, "Adam Data In"=w56) -> ("Output"=w40:dbl, "Error"=w46:dbl, "Adjusted Parameters"=w44:T4, "Adam Data Out"=w57:T2)  [unwired: 4 in, 1 out]
    "NN Output" <- w40
    "NN Error" <- w46
    "NN Loss" <- w46
    n492 = Subtract(x=4, y=w108) -> (x-y=w105:dbl)
    n493 = call "Signal Production.vi"("Polarization"=w40) -> ("output cluster"=→"NN Graph":cluster{dbl[], "result":dbl[]})  [unwired: 10 in]
    n494 = Square Root(x=w105) -> (sqrt(x)=w110:dbl)
    n495 = Less?(x=w47, y=w46) -> (x < y?=w45:bool)
    n496 = Subtract(x=2, y=w110) -> ()  [unwired: 1 out]
    n497 = Select(t=w47, s=w45, f=w46) -> (s? t:f=w48:dbl)
    n498 = Select(t=w42, s=w45, f=w44) -> (s? t:f=w43:T4)
  }
  n499 = invoke class="VI" method="Default Vals.Reinit All"(reference=w38) -> ()  [unwired: 2 in, 3 out]
  n500 = property on="Total Polarization (P)" class="WFChart (strict)"("History Data"=cluster{dbl, dbl}[] []) -> ()  [unwired: 2 in, 2 out]
  n501 = property on="NN Training Loss" class="WFChart (strict)"("History Data"=dbl[] []) -> ()  [unwired: 2 in, 2 out]
  n502 = Close File(refnum=w34, error in=w33) -> ()  [unwired: 2 out]
  n503 = Flatten To XML(6:w2) -> (2:w30:string)
  n504 = call-poly <vilib>:"Write to XML File.vi"("XML Input"=w30, "XML File Path"="Parameters File Path") -> ()  [unwired: 7 in, 3 out]
